vi "Read Alarm Options.vi"(0 "VISA resource name":refnum<visa-resource-name>, 5 "error in (no error)":errorcluster) -> (10 "Input Alarm":bool, 12 "Output of Input Alarm":bool, 13 "Output of the Auto Increment Alarm":bool, 14 "VISA resource name out":refnum<visa-resource-name>, 15 "Latch the Input Alarm":bool, 16 "Output of the Pressure Alarm":bool, 17 "Latch the Pressure Alarm":bool, 18 "Auto Increment Alarm":bool, 19 "error out":errorcluster)   [LabVIEW 2020, in "EFD Ultimus V.lvlib"]
doc: "Reads the current settings of the alarm options in the Ultimus V."
uses:
  EFD Ultimus V.lvlib
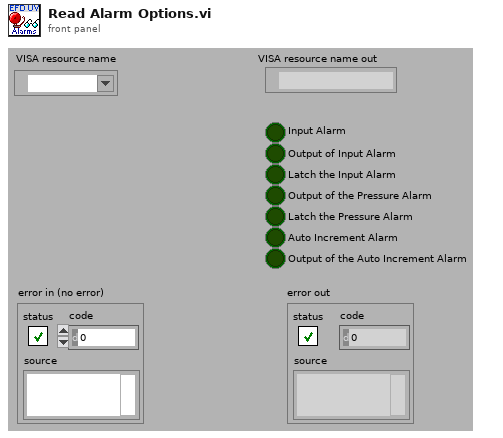
[diagram p1: front panel]
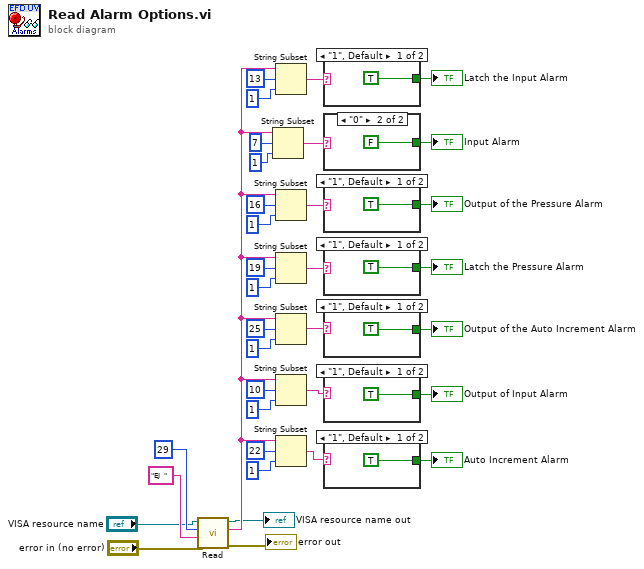
[diagram p0: block diagram]
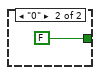
[diagram p2: hidden frame]
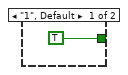
[diagram p3: hidden frame]
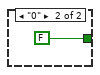
[diagram p4: hidden frame]
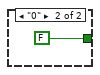
[diagram p5: hidden frame]
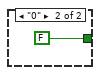
[diagram p6: hidden frame]
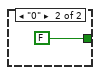
[diagram p7: hidden frame]
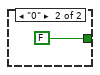
[diagram p8: hidden frame]
diagram:
  n1 = call "Read.vi"("error in (no error)"="error in (no error)", "Command To Write"="EJ  ", "Bytes to Read (11)"=u32 29 ("Bytes to Read from Buffer"), "VISA resource name"="VISA resource name") -> ("error out"=→"error out":errorcluster, "Ultimus V Feedback Data"=w5:string, "VISA resource name out"=→"VISA resource name out":refnum<visa-resource-name>)  [unwired: 5 out]
  n2 = String Subset(string=w5, offset (0)=7, length (rest)=1 ("length (rest)")) -> (substring=w34:string)
  n3 = String Subset(string=w5, offset (0)=13, length (rest)=1 ("length (rest)")) -> (substring=w22:string)
  n4 = String Subset(string=w5, offset (0)=16, length (rest)=1 ("length (rest)")) -> (substring=w30:string)
  n5 = String Subset(string=w5, offset (0)=19, length (rest)=1 ("length (rest)")) -> (substring=w31:string)
  n6 = String Subset(string=w5, offset (0)=25, length (rest)=1 ("length (rest)")) -> (substring=w33:string)
  n7 = String Subset(string=w5, offset (0)=10, length (rest)=1 ("length (rest)")) -> (substring=w35:string)
  n8 = String Subset(string=w5, offset (0)=22 ("length (rest)"), length (rest)=1 ("length (rest)")) -> (substring=w32:string)
  n9 = case shown="\"1\", Default" w22 {
    tunnel: [TRUE ("Latch the Input Alarm") FALSE ("Latch the Input Alarm")] -> w23
    frame "1", Default {
    }
    frame "0" {
    }
  }
  "Latch the Input Alarm" <- w23
  n10 = case shown="\"0\"" w34 {
    tunnel: [TRUE ("Latch the Input Alarm") FALSE ("Latch the Input Alarm")] -> w28
    frame "1", Default {
    }
    frame "0" {
    }
  }
  "Input Alarm" <- w28
  n11 = case shown="\"1\", Default" w30 {
    tunnel: [TRUE ("Latch the Input Alarm") FALSE ("Latch the Input Alarm")] -> w24
    frame "1", Default {
    }
    frame "0" {
    }
  }
  "Output of the Pressure Alarm" <- w24
  n12 = case shown="\"1\", Default" w31 {
    tunnel: [TRUE ("Latch the Input Alarm") FALSE ("Latch the Input Alarm")] -> w25
    frame "1", Default {
    }
    frame "0" {
    }
  }
  "Latch the Pressure Alarm" <- w25
  n13 = case shown="\"1\", Default" w33 {
    tunnel: [TRUE ("Latch the Input Alarm") FALSE ("Latch the Input Alarm")] -> w27
    frame "1", Default {
    }
    frame "0" {
    }
  }
  "Output of the Auto Increment Alarm" <- w27
  n14 = case shown="\"1\", Default" w35 {
    tunnel: [TRUE ("Latch the Input Alarm") FALSE ("Latch the Input Alarm")] -> w29
    frame "1", Default {
    }
    frame "0" {
    }
  }
  "Output of Input Alarm" <- w29
  n15 = case shown="\"1\", Default" w32 {
    tunnel: [TRUE ("Latch the Input Alarm") FALSE ("Latch the Input Alarm")] -> w26
    frame "1", Default {
    }
    frame "0" {
    }
  }
  "Auto Increment Alarm" <- w26
